vi "sdh_word_table.vi"() -> ()   [LabVIEW 2018]
uses:
  <vilib>/Utility/NIReport.llb/Report Type.ctl
  <vilib>/addons/_office/_exclsub.llb/font.ctl
  <vilib>/addons/_office/word.llb/Word Easy Table (str).vi
  <vilib>/Utility/NIReport.llb/NI_report.lvclass
  <vilib>/Utility/NIReport.llb/NI_ReportGenerationCore.lvlib
  <vilib>/addons/_office/NI_ReportGenerationToolkit.lvlib
panel:
  in  "添加的数组":string[][](array[string])
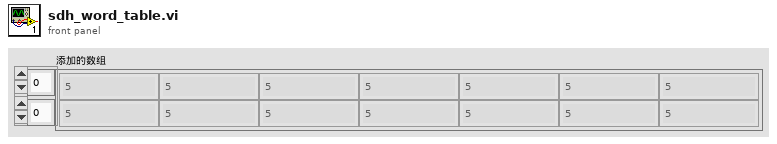
[diagram p1: front panel]
types:
  T1 = typedef "NI_ReportGenerationToolkit.lvlib/font.ctl" = cluster{"font name":string, "font size":dbl, "bold":u16, "italic":u16, "underline":u16, "strike through":u16, "font color":u32}
  T2 = enum16{"maximized", "minimized", "normal", "no change"}
  T3 = typedef "NI_ReportGenerationCore.lvlib/Report Type.ctl" = enum16{"HTML", "Word", "Excel"}
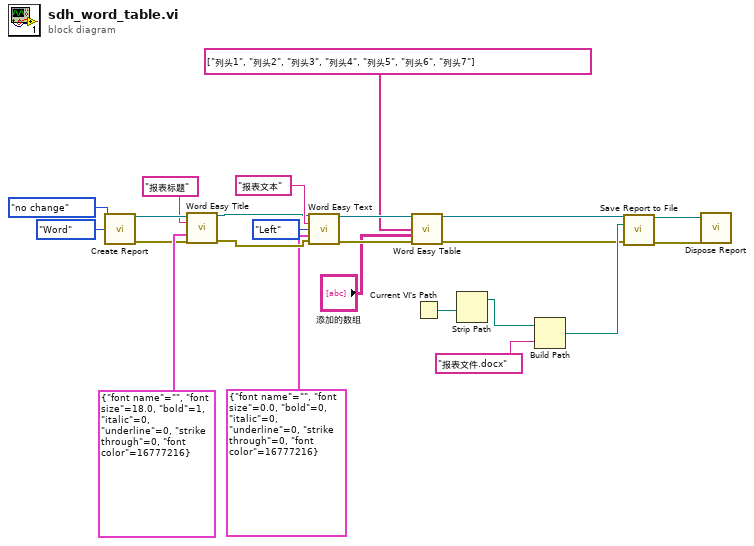
[diagram p0: block diagram]
diagram:
  n1 = call <vilib>:"Create Report.vi"("window state (normal)"=T2."no change", "report type"=Report_Type."Word") -> ("report out"=w18:refnum<class "NI_report.lvclass">, "error out"=w14:errorcluster)  [unwired: 12 in]
  n2 = call <vilib>:"Word Easy Title.vi"("report in"=w18, "title"="报表标题", "font"=T1 {"font name"="", "font size"=18.0, "bold"=1, "italic"=0, "underline"=0, "strike through"=0, "font color"=16777216}, "error in (no error)"=w14) -> ("report out"=w8:refnum<class "NI_report.lvclass">, "error out"=w13:errorcluster)  [unwired: 9 in, 1 out]
  n3 = call <vilib>:"Word Easy Text.vi"("report in"=w8, "text"="报表文本", "alignment (left)"=enum16{"Left", "Centered", "Right", "Justify"}."Left", "font"=T1 {"font name"="", "font size"=0.0, "bold"=0, "italic"=0, "underline"=0, "strike through"=0, "font color"=16777216}, "error in (no error)"=w13) -> ("report out"=w9:refnum<class "NI_report.lvclass">, "error out"=w10:errorcluster)  [unwired: 8 in, 1 out]
  n4 = call-poly <vilib>:"Word Easy Table.vi"("report in"=w9, "column headers"=string[] ["列头1", "列头2", "列头3", "列头4", "列头5", "列头6", "列头7"], "data"="添加的数组", "error in (no error)"=w10) -> ("report out"=w6:refnum<class "NI_report.lvclass">, "error out"=w2:errorcluster)  [unwired: 9 in, 1 out]
  n5 = Current VI's Path() -> (path=w23:path)
  n6 = Strip Path(path=w23) -> (stripped path=w22:path)  [unwired: 1 out]
  n7 = Build Path(base path=w22, name or relative path="报表文件.docx" ("名称或相对路径")) -> (appended path=w5:path)
  n8 = call-dynamic "Save Report to File.vi"("report in"=w6, "report file path"=w5, "error in (no error)"=w2) -> ("report out"=w4:refnum<class "NI_report.lvclass">, "error out"=w3:errorcluster)  [unwired: 11 in]
  n9 = call-dynamic "Dispose Report.vi"("report in"=w4, "error in (no error)"=w3) -> ()  [unwired: 13 in, 1 out]
